vi "Send Omni Packet.vi"(11 "output cluster":T1) -> ()   [LabVIEW 2013]
uses:
  Common Code/Dashboard UDP/Omni Packet.ctl
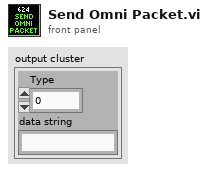
[diagram p1: front panel]
types:
  T1 = typedef "Omni Packet.ctl" = cluster{"Type":i32, "data string":string}
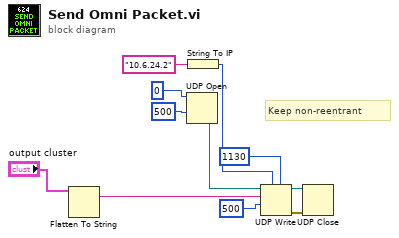
[diagram p0: block diagram]
diagram:
  # "Keep non-reentrant"
  n1 = Flatten To String(anything="output cluster") -> (data string=w2:string)  [unwired: 3 in, 2 out]
  n2 = UDP Open(9:500 ("timeout ms (25000)"), 11:u16 0 ("port")) -> (port=w9:refnum<k16>)  [unwired: 3 in, 2 out]
  n3 = String To IP(1:"10.6.24.2" ("name")) -> (0:w5:u32)
  n4 = UDP Write(address=w5, port or service name=u16 1130 ("port"), connection ID=w9, data in=w2, 9:500 ("timeout ms (25000)")) -> (error out=w10:errorcluster, 3:w11:refnum<k16>)  [unwired: 1 in]
  n5 = UDP Close(connection ID=w11, 8:w10) -> ()  [unwired: 2 out]
